vi "Tower Bar Drop Ropes Logic.vi"(11 "Input":dbl) -> ()   [LabVIEW 2016]
uses:
  <vilib>/Rock Robotics/Network Tables/NT Read Boolean.vi
  Robot Global Data.vi
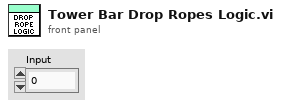
[diagram p1: front panel]
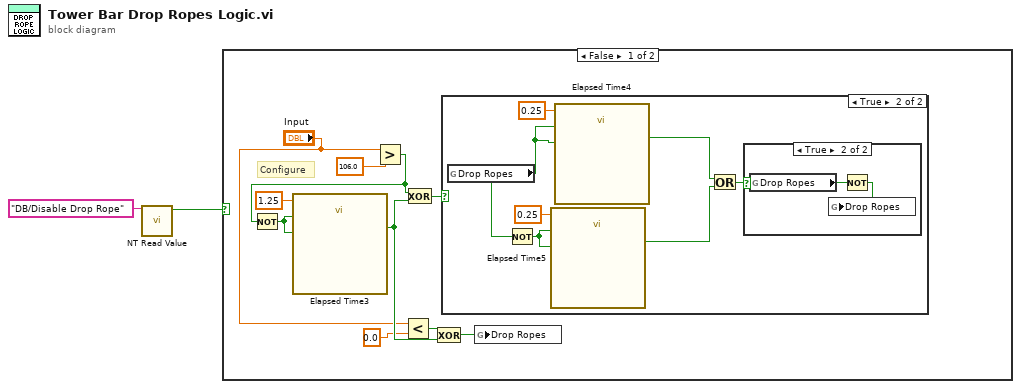
[diagram p0: block diagram]
diagram:
  n1 = call-poly <vilib>:"NT Read Value.vi"("Name"="DB/Disable Drop Rope") -> ("Boolean"=w2:bool)  [unwired: 9 in, 1 out]
  n2 = case shown="False" w2 {
    frame False {
      # "Configure"
      n3 = Greater?(x="Input", y=106.0) -> (0:w9:bool)
      n4 = Not(x=w9) -> (.not. x?=w12:bool)
      n5 = call "Elapsed Time3"("Time Target (s)"=1.25, "Reset"=w12, "Auto Reset"=w12) -> ("Time has Elapsed"=w7:bool)  [unwired: 9 in, 7 out]
      n6 = Less?(x="Input", y=0.0) -> (x < y?=w5:bool)
      n7 = Exclusive Or(1:w7, 2:w9) -> (0:w8:bool)
      n8 = Exclusive Or(1:w7, 2:w5) -> (0:w6:bool)
      n9 = case shown="True" w8 {
        frame False {
        }
        frame True {
          n10 = global read "Robot Global Data.vi" "Drop Ropes"() -> (w13:bool)
          n11 = Not(x=w13) -> (.not. x?=w14:bool)
          n12 = call "Elapsed Time5"("Time Target (s)"=0.25, "Reset"=w14, "Auto Reset"=w14) -> ("Time has Elapsed"=w15:bool)  [unwired: 9 in, 7 out]
          n13 = call "Elapsed Time4"("Time Target (s)"=0.25, "Reset"=w13, "Auto Reset"=w13) -> ("Time has Elapsed"=w16:bool)  [unwired: 9 in, 7 out]
          n14 = Or(x=w16, y=w15) -> (x .or. y?=w17:bool)
          n15 = case shown="True" w17 {
            frame False {
            }
            frame True {
              n16 = global read "Robot Global Data.vi" "Drop Ropes"() -> (w21:bool)
              n17 = Not(x=w21) -> (.not. x?=w20:bool)
              n18 = global write "Robot Global Data.vi" "Drop Ropes"(w20) -> ()
            }
          }
        }
      }
      n19 = global write "Robot Global Data.vi" "Drop Ropes"(w6) -> ()
    }
    frame True {
    }
  }
